vi "Stop Core.vi"(10 "final error code":i32, 11 "Fluke Hydra 2625A in":refnum<class "Fluke Hydra 2625A.lvclass">) -> (3 "Fluke Hydra 2625A out":refnum<class "Fluke Hydra 2625A.lvclass">)   [LabVIEW 2014, in "Generic Data Acquisition.lvlib" / "Fluke Hydra.lvlib" / "Fluke Hydra 2625A.lvclass"]
doc: "(<B>Filename</B>: Actor Framework.lvlib:Actor.lvclass:Stop Core.vi)\n\nDefines what the actor does before it stops. Use the <B>final error code</B> input to determine whether the actor shut down in response to an error.\n\nBy default, this method does nothing. A descendant class may override it to define behavior, such as shutting down any processes the actor initiated in its override of the Actor Core method."
uses:
  Fluke Hydra 2625A.lvclass
  Generic Data Acquisition.lvclass
  <instrlib>/Fluke 2625A/Fluke 2625A.lvlib
panel:
  out "Error Out":errorcluster
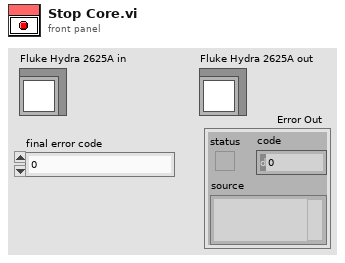
[diagram p1: front panel]
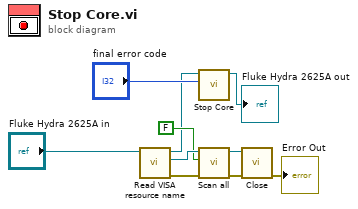
[diagram p0: block diagram]
diagram:
  n1 = call-dynamic "Read VISA resource name.vi"("Generic Instrument in"="Fluke Hydra 2625A in") -> ("error out"=w6:errorcluster, "VISA resource name"=w8:refnum<visa-resource-name>, "Generic Instrument out"=w2:refnum<class "Fluke Hydra 2625A.lvclass">)  [unwired: 8 in]
  n2 = call-parent "Stop Core.vi"("final error code"="final error code", "Generic Instrument in"=w2) -> ("Generic Instrument out"=→"Fluke Hydra 2625A out":refnum<class "Fluke Hydra 2625A.lvclass">)  [unwired: 9 in]
  n3 = call <instrlib>:"Scan all.vi"("Error In"=w6, "Start/Stop In"=FALSE, "VISA Resource Name In"=w8) -> ("Error Out"=w5:errorcluster, "VISA Resource Name Out"=w7:refnum<visa-resource-name>)  [unwired: 6 in, 1 out]
  n4 = call <instrlib>:"Close.vi"("Error In"=w5, "VISA Resource Name In"=w7) -> ("Error Out"=→"Error Out":errorcluster)  [unwired: 9 in]
